vi "WindowAdjust.vi"(8 "error in (no error)":errorcluster, 11 "Fitter in":refnum<class "FitterBase.lvclass">) -> (0 "error out":errorcluster, 2 "SamplesNeeded":u32, 3 "Fitter out":refnum<class "FitterBase.lvclass">)   [LabVIEW 2018, in "AnalysisPlugins.lvlib" / "FitterBase.lvclass"]
uses:
  FitterBaseClass/FitterBase.lvclass
  C:/projects/ICDAS/NistPluggableModules/Analysis/AnalysisPlugins/AnalysisPluginBaseClass/AnalysisPluginsBase.lvclass
  FitterBaseClass/Typedefs/clAnalysisConfig.ctl
  AnalysisPluginsBase.lvclass/AnalysisPluginsBase.ctl
  Accessors/Read AnalysisTime.vi
  Accessors/Read Window.vi
  Accessors/Read AnalysisConfig.vi
  Accessors/Write Window.vi
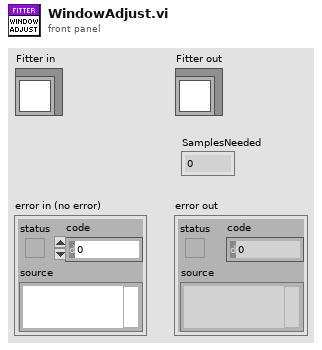
[diagram p1: front panel]
types:
  T1 = typedef "AnalysisPlugins.lvlib/FitterBase.lvclass/clAnalysisConfig.ctl" = cluster{"F0":u32, "SettlingTime":dbl, "AnalysisCycles":dbl, "SampleRate":dbl, "NumChannels":u32, "TsOffset":enum16{"start", "middle", "end"}}
  T2 = typedef "AnalysisPlugins.lvlib/AnalysisPluginsBase.lvclass/clWindowData.ctl" = cluster{"Timestamp":ext, "Samples":dbl[][], "Window Valid":bool, "T0":ext}
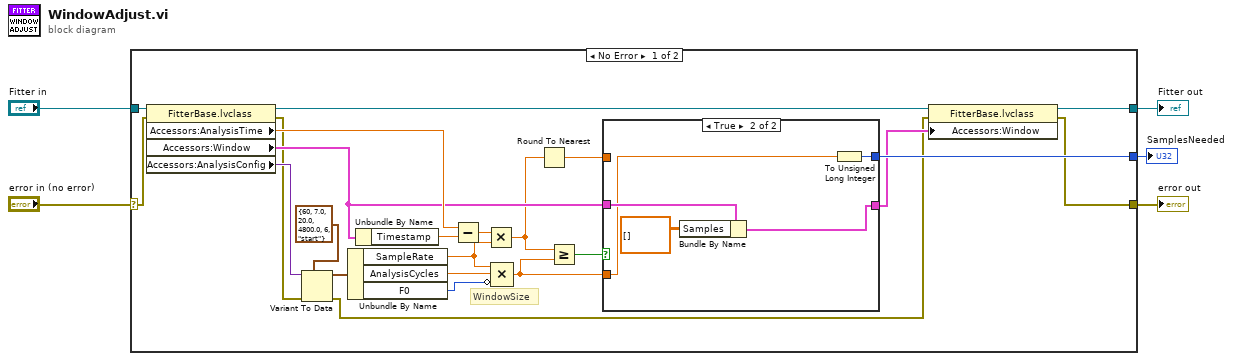
[diagram p0: block diagram]
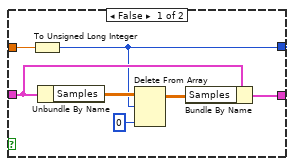
[diagram p2: hidden frame]
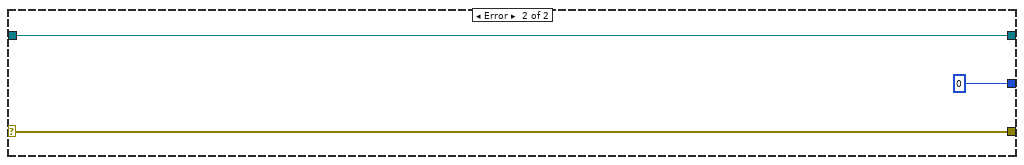
[diagram p3: hidden frame]
diagram:
  n1 = case shown="No Error" "error in (no error)" {
    selector: "error in (no error)" -> [w7 w43]
    tunnel: [w6 w43] -> w4
    tunnel: [w16 w42] -> w2
    tunnel: "Fitter in" -> [w28 w42]
    tunnel: [w17 u32 0] -> w1
    frame No Error {
      # "WindowSize"
      n2 = property class="FitterBase.lvclass"(reference=w28, error in=w7) -> (reference out=w27:refnum<class "FitterBase.lvclass">, error out=w9:errorcluster, "Accessors:AnalysisTime"=w25:dbl, "Accessors:Window"=w19:T2, "Accessors:AnalysisConfig"=w12:variant)
      n3 = Variant To Data(error in=w9, type=T1 {"F0"=60, "SettlingTime"=7.0, "AnalysisCycles"=20.0, "SampleRate"=4800.0, "NumChannels"=6, "TsOffset"=enum."start"} ("clAnalysisConfig"), Variant=w12) -> (data=w10:T1, error out=w8:errorcluster)
      n4 = Unbundle By Name(w10) -> ("SampleRate"=w23:dbl, "AnalysisCycles"=w22:dbl, "F0"=w21:u32)
      n5 = Unbundle By Name(w19) -> ("Timestamp"=w26:ext)
      n6 = Subtract(x=w25, y=w26) -> (x-y=w24:ext)
      n7 = Multiply(x=w24, y=w23) -> (x*y=w18:ext)
      n8 = Compound Arithmetic op=MULTIPLY(w23, w22, invert w21) -> (w14:dbl)
      n9 = Round To Nearest(number=w18) -> (nearest integer value=w13:ext)
      n10 = Greater Or Equal?(x=w18, y=w14) -> (x >= y?=w20:bool)
      n11 = case shown="True" w20 {
        tunnel: w19 -> [w32 w40]
        tunnel: [w29 w36] -> w17
        tunnel: [w31 w38] -> w15
        tunnel: w14 -> [_ w37]
        tunnel: w13 -> [w30 _]
        frame False {
          n12 = To Unsigned Long Integer(number=w30) -> (unsigned 32bit integer=w29:u32)
          n13 = Unbundle By Name(w32) -> ("Samples"=w35:dbl[][])
          n14 = Delete From Array(array=w35, length=w29, index (col)=0 ("disabled index (col)")) -> (array with subset deleted=w33:dbl[][])  [unwired: 1 in, 1 out]
          n15 = Bundle By Name(cluster=w32, "Samples"=w33) -> (w31:T2)
        }
        frame True {
          n16 = Bundle By Name(cluster=w40, "Samples"=dbl[][] []) -> (w38:T2)
          n17 = To Unsigned Long Integer(number=w37) -> (unsigned 32bit integer=w36:u32)
        }
      }
      n18 = property class="FitterBase.lvclass"(reference=w27, error in=w8, "Accessors:Window"=w15) -> (reference out=w16:refnum<class "FitterBase.lvclass">, error out=w6:errorcluster)
    }
    frame Error {
    }
  }
  "error out" <- w4
  "Fitter out" <- w2
  "SamplesNeeded" <- w1
